vi "CH_LM Test Streaming.vi"() -> ()   [LabVIEW 2012, in "CH_LM.lvlib"]
doc: "This example VI starts the data acquisition and displays the measured data."
uses:
  CH_LM.lvlib
  CH_LM/CH_LM Streaming Data.ctl
  CH_LM/CH_LM Data Token.ctl
  CH_LM/CH_LM Measurement Delivery Mode.ctl
  CH_LM/CH_LM BaudRates.ctl
  CH_LM/CH_LM Parity.ctl
  CH_LM/CH_LM SerialConfiguration.ctl
panel:
  out "dt / ms":u32
  out "size":i32
  in  "Serial Configuration\n(19200,N,8,1)":T1={"Baud Rate"=19200, "Parity"=0, "Data Bits"=8, "Stop Bits"=1} {"Parity" items=["None", "Odd", "Even"]; "Baud Rate" items=["9600"=9600, "19200"=19200, "38400"=38400, "57600"=57600, "115200"=115200]}
  in  "Delivery Mode":T4=enum."Stream"
  in  "ID Query? (T: Yes)":bool
  in  "Reset? (F: No)":bool
  in  "Serial Number":string
  in  "Address":i32=1
  out "Data OK":bool
  out "Steaming Data Cluster":T5 {"Flags" format="%.0b"; "Unit ID" format="%.0b"; "Quad Distance"."Y" format="%#.1f"; "Quad Distance"."X" format="%#.1f"; "Value" format="%#.7e"}
  out "Data Header":bool
  in  "stopp":bool
  out "Data Tokens":T6[](array[typedef])=[enum."Raw data"]
  out "Stream error":errorcluster
  in  "Reset":bool
  out "Steaming Data Chart":T7(graph)
  out "timed out?":bool
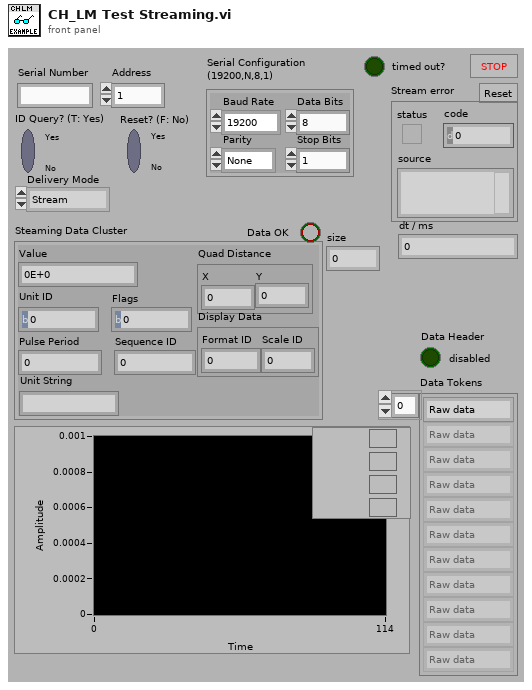
[diagram p1: front panel]
types:
  T1 = typedef "CH_LM.lvlib/CH_LM SerialConfiguration.ctl" = cluster{"Baud Rate":T2, "Parity":T3, "Data Bits":u16, "Stop Bits":u16}
  T2 = typedef "CH_LM.lvlib/CH_LM BaudRates.ctl" = u32
  T3 = typedef "CH_LM.lvlib/CH_LM Parity.ctl" = u16
  T4 = typedef "CH_LM.lvlib/CH_LM Measurement Delivery Mode.ctl" = enum16{"Last", "Stream"}
  T5 = typedef "CH_LM.lvlib/CH_LM Streaming Data.ctl" = cluster{"Value":sgl, "Quad Distance":cluster{"X":sgl, "Y":sgl}, "Display Data":cluster{"Format ID":u8, "Scale ID":u8}, "Unit ID":u8, "Flags":u32, "Pulse Period":u32, "Sequence ID":u32, "Unit String":string}
  T6 = typedef "CH_LM.lvlib/CH_LM Data Token.ctl" = enum16{"Raw data", "Quad distance", "Formated data", "Unit", "Pulse period", "Flags", "Sequence ID"}
  T7 = cluster{"Value":sgl, "X":sgl, "Y":sgl, "Pulse Period":u32}[]
  T8 = cluster{"Value":sgl, "X":sgl, "Y":sgl, "Pulse Period":u32}
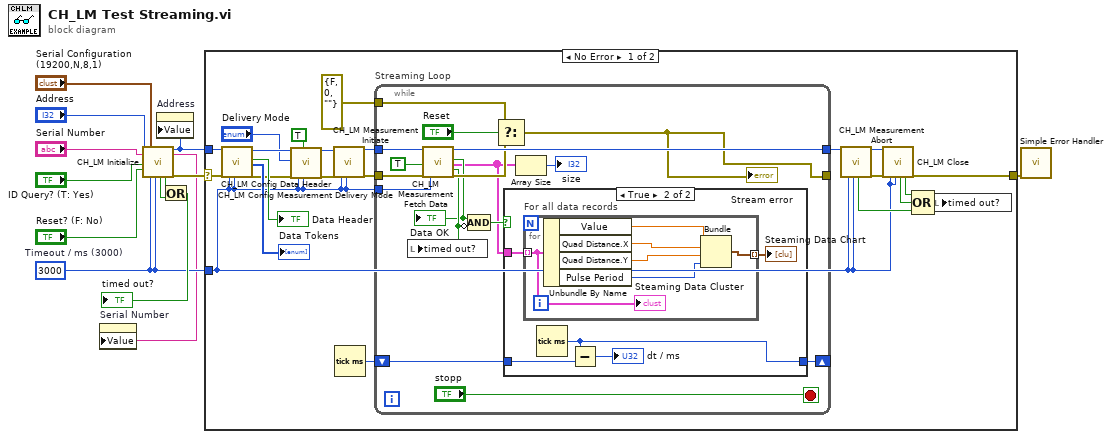
[diagram p0: block diagram]
diagram:
  w8 = 3000  # Timeout / ms (3000)
  n1 = call "CH_LM Initialize.vi"("Address"="Address", "Serial Number"="Serial Number", "ID Query (True)"="ID Query? (T: Yes)", "Reset (False)"="Reset? (F: No)", "Serial Configuration\n(19200,N,8,1)"="Serial Configuration\n(19200,N,8,1)", "Timeout / ms (3000)"=w8, "Lock Timeout / ms (1000)"=w8) -> ("Lock timed out"=w10:bool, "timed out?"=w11:bool, "Meter Index"=w2:i32, "Serial Number"=w1:string, "error out"=w7:errorcluster)  [unwired: 1 in, 7 out]
  n2 = property on="Serial Number" class="Str"("Value"=w1) -> ()  [unwired: 2 in, 2 out]
  n3 = property on="Address" class="DigNum (strict)"("Value"=w2) -> ()  [unwired: 2 in, 2 out]
  n4 = Or(x=w11, y=w10) -> (x .or. y?=→"timed out?":bool)
  n5 = case shown="No Error" w7 {
    selector: w7 -> [w27 w66]
    tunnel: w2 -> [w36 _]
    tunnel: w8 -> [w17 _]
    tunnel: [w14 w66] -> w4
    frame No Error {
      n6 = call "CH_LM Config Data Header.vi"("Meter Index"=w36, "error in (no error)"=w27, "Timeout / ms (3000)"=w17, "Lock Timeout / ms (1000)"=w17) -> ("Meter Index"=w20:i32, "Data Header"=→"Data Header":bool, "Data Tokens"=→"Data Tokens":T6[], "error out"=w19:errorcluster)  [unwired: 3 in, 9 out]
      n7 = call "CH_LM Config Measurement Delivery Mode.vi"("Meter Index"=w20, "Delivery Mode"="Delivery Mode", "error in (no error)"=w19, "Timeout / ms (3000)"=w17, "Action (query)"=TRUE, "Lock Timeout / ms (1000)"=w17) -> ("Meter Index"=w21:i32, "error out"=w18:errorcluster)  [unwired: 12 out]
      n8 = call "CH_LM Measurement Initiate.vi"("Meter Index"=w21, "error in (no error)"=w18, "Timeout / ms (3000)"=w17, "Lock Timeout / ms (1000)"=w17) -> ("Meter Index"=w33:i32, "error out"=w31:errorcluster)  [unwired: 14 out]
      n9 = Tick Count (ms)() -> (millisecond timer value=w29:u32)
      n10 = while "Streaming Loop" {
        tunnel: w33 -> [w53]
        tunnel: [w52] -> w32
        tunnel: w17 -> [w51]
        tunnel: errorcluster {"status"=FALSE, "code"=0, "source"=""} ("error in (no error)") -> [w49]
        shift-right: [w46] -> _
        shift-left: w29 -> [w47]
        tunnel: w31 -> [w43]
        tunnel: [w45] -> _
        stop <- "stopp" stop-if-true
        n11 = call "CH_LM Measurement Fetch Data.vi"("Meter Index"=w53, "All Records? (F)"=TRUE, "error in (no error)"=w43, "Timeout / ms (1000)"=w51) -> ("Meter Index"=w52:i32, "Data OK"=w41:bool, "Data Array"=w38:T5[], "timed out?"=w42:bool, "error out"=w48:errorcluster)  [unwired: 1 in, 10 out]
        "Data OK" <- w41
        n12 = local write "timed out?"(w42) -> ()
        n13 = Compound Arithmetic op=AND(w41, invert w42) -> (w40:bool)
        n14 = Select(t=w49, s="Reset", f=w48) -> (s? t:f=w45:errorcluster)
        "Stream error" <- w45
        n15 = case shown="True" w40 {
          tunnel: w38 -> [_ w59]
          tunnel: w47 -> [w54 w58]
          tunnel: [w54 w57] -> w46
          frame False {
          }
          frame True {
            n16 = for "For all data records" {
              tunnel: w59 -> [w65] mode=indexing
              tunnel: [w63] -> w56 mode=indexing
              n17 = Unbundle By Name(w65) -> ("Value"=w64:sgl, "Quad Distance.X"=w62:sgl, "Quad Distance.Y"=w61:sgl, "Pulse Period"=w60:u32)
              n18 = Bundle("Value"=w64, "X"=w62, "Y"=w61, "Pulse Period"=w60) -> (w63:T8)  [unwired: 1 out]
              "Steaming Data Cluster" <- w65
            }
            "Steaming Data Chart" <- w56
            n19 = Tick Count (ms)() -> (millisecond timer value=w57:u32)
            n20 = Subtract(x=w57, y=w58) -> (x-y=→"dt / ms":u32)
          }
        }
        n21 = Array Size(array=w38) -> (size(s)=→"size":i32)
      }
      n22 = call "CH_LM Measurement Abort.vi"("Meter Index"=w32, "Timeout / ms (3000)"=w17, "Lock Timeout / ms (1000)"=w17) -> ("Lock timed out"=w25:bool, "Meter Index"=w34:i32, "error out"=w35:errorcluster)  [unwired: 1 in, 13 out]
      n23 = call "CH_LM Close.vi"("Meter Index"=w34, "error in (no error)"=w35, "Timeout / ms (3000)"=w17, "Lock Timeout / ms (1000)"=w17) -> ("Lock timed out"=w23:bool, "timed out?"=w24:bool, "error out"=w14:errorcluster)  [unwired: 13 out]
      n24 = Compound Arithmetic op=OR(w24, w23, w25) -> (w22:bool)
      n25 = local write "timed out?"(w22) -> ()
    }
    frame Error {
    }
  }
  n26 = call <vilib>:"Simple Error Handler.vi"("error in (no error)"=w4) -> ()  [unwired: 1 in, 8 out]
